vi "trio_test.vi"() -> ()   [LabVIEW 2017]
uses:
  <instrlib>/Trio Motion/Trio Motion Library.lvlib
panel:
  out "Reverse Limit":bool
  out "Forward Limit":bool
  in  "Distance":dbl format="%#_13g"
  in  "Move rel":bool
  in  "Axis":i16
  in  "Variable":string="MPOS"
  out "Value":dbl=-1.0 format="%#_13g"
  out "error out":errorcluster
  in  "stop":bool
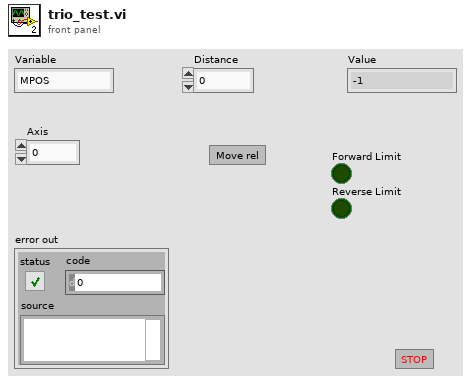
[diagram p1: front panel]
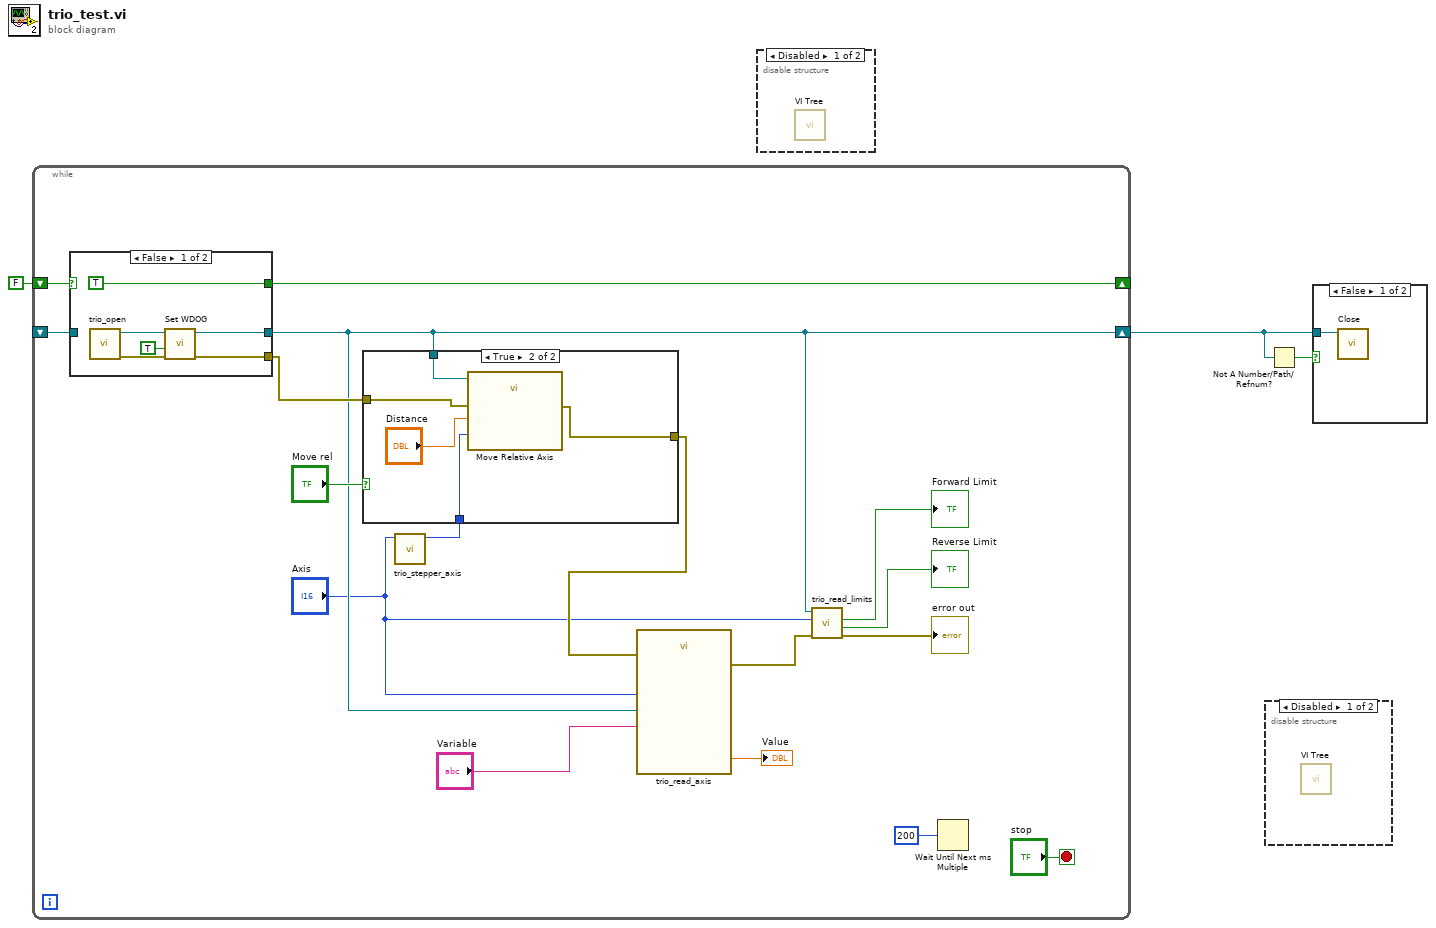
[diagram p0: block diagram]
diagram:
  n1 = while {
    shift-right: [w18] -> _
    shift-left: FALSE -> [w19]
    shift-right: [w9] -> w3
    shift-left: _ -> [w17]
    stop <- "stop" stop-if-true
    n2 = case shown="False" w19 {
      selector: w19 -> [_ w33]
      tunnel: [TRUE w33] -> w18
      tunnel: [w27 w34] -> w9
      tunnel: w17 -> [_ w34]
      tunnel: [w28 _] -> w12
      frame False {
        n3 = call "trio_open.vi"() -> ("error out"=w30:errorcluster, "reference out"=w29:refnum<k7>)  [unwired: 10 in]
        n4 = call <instrlib>:"Set WDOG.vi"("error in (no error)"=w30, "WDOG (ON)"=TRUE, "reference in"=w29) -> ("error out"=w28:errorcluster, "reference out"=w27:refnum<k7>)  [unwired: 6 in, 1 out]
      }
      frame True {
      }
    }
    n5 = call "trio_stepper_axis.vi"("Encoder axis"="Axis") -> ("Stepper axis"=w7:i32)  [unwired: 10 in]
    n6 = case shown="True" "Move rel" {
      tunnel: w9 -> [_ w25]
      tunnel: w12 -> [w21 w24]
      tunnel: [w21 w23] -> w11
      tunnel: w7 -> [_ w22]
      frame False {
      }
      frame True {
        n7 = call <instrlib>:"Move Relative Axis.vi"("error in (no error)"=w24, "Distance"="Distance", "Axis (0)"=w22, "reference in"=w25) -> ("error out"=w23:errorcluster)  [unwired: 5 in, 2 out]
      }
    }
    n8 = call "trio_read_axis.vi"("Axis"="Axis", "error in (no error)"=w11, "Variable"="Variable", "reference in"=w9) -> ("error out"=w8:errorcluster, "Value"=→"Value":dbl)  [unwired: 5 in, 1 out]
    n9 = call "trio_read_limits.vi"("error in (no error)"=w8, "Axis"="Axis", "Trio ref in"=w9) -> ("error out"=→"error out":errorcluster, "Reverse Limit"=→"Reverse Limit":bool, "Forward Limit"=→"Forward Limit":bool)  [unwired: 5 in, 1 out]
    n10 = Wait Until Next ms Multiple(millisecond multiple=u32 200) -> ()  [unwired: 1 out]
  }
  n11 = disable-structure shown="Disabled" {
    frame Disabled {
      n12 = call <instrlib>:"VI Tree.vi"() -> ()  [unwired: 12 in]
    }
    frame Enabled {
    }
  }
  n13 = disable-structure shown="Disabled" {
    frame Disabled {
      n14 = call <instrlib>:"VI Tree.vi"() -> ()  [unwired: 12 in]
    }
    frame Enabled {
    }
  }
  n15 = Not A Number/Path/Refnum?(number/path/refnum=w3) -> (NaN/Path/Refnum?=w2:bool)
  n16 = case shown="False" w2 {
    tunnel: w3 -> [w35 _]
    frame False {
      n17 = call <instrlib>:"Close.vi"("reference in"=w35) -> ()  [unwired: 10 in, 1 out]
    }
    frame True {
    }
  }
